vi "utility_edit_device_tree_items_02_01.vi"() -> ()   [LabVIEW 2015]
panel:
  in  "device tree":string[](tree)=["FCXF-X-03-S05"] caption="设备列表"
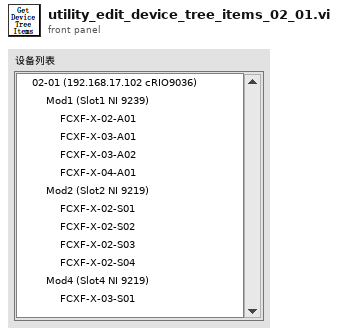
[diagram p1: front panel]
types:
  T1 = enum16{"open", "replace", "create", "open or create", "replace or create", "replace or create with confirmation"}
  T2 = cluster{"Left Cell String":string, "Child Text":string[], "Child Tag":string, "Item Indent":i32, "Child Only?":bool, "Glyph Index":i32}
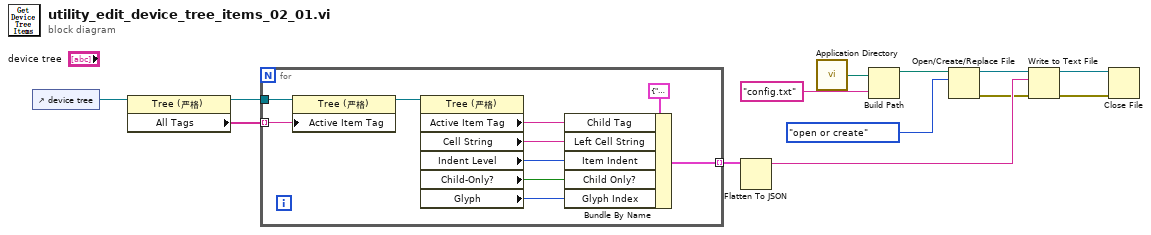
[diagram p0: block diagram]
diagram:
  n1 = control-ref of="device tree"() -> (w13:refnum<vi>)
  n2 = property class="Tree (严格)"(reference=w13) -> (reference out=w12:refnum<vi>, "All Tags"=w11:string[])  [unwired: 1 in, 1 out]
  n3 = for {
    tunnel: w12 -> [w23]
    tunnel: w11 -> [w21] mode=indexing
    tunnel: [w14] -> w10 mode=indexing
    n4 = property class="Tree (严格)"(reference=w23, "Active Item Tag"=w21) -> (reference out=w22:refnum<vi>)  [unwired: 1 in, 1 out]
    n5 = property class="Tree (严格)"(reference=w22) -> ("Active Item Tag"=w19:string, "Cell String"=w18:string, "Indent Level"=w17:i32, "Child-Only?"=w16:bool, "Glyph"=w15:i32)  [unwired: 1 in, 2 out]
    n6 = Bundle By Name(cluster=T2 {"Left Cell String"="FCXF-X-03-T02", "Child Text"=[], "Child Tag"="FCXF-X-03-T02", "Item Indent"=2, "Child Only?"=TRUE, "Glyph Index"=4} ("Item"), "Child Tag"=w19, "Left Cell String"=w18, "Item Indent"=w17, "Child Only?"=w16, "Glyph Index"=w15) -> (w14:T2)
  }
  n7 = Flatten To JSON(anything=w10) -> (JSON string=w9:string)  [unwired: 2 in, 1 out]
  n8 = call <vilib>:"Application Directory.vi"() -> ("Application Directory"=w4:path)
  n9 = Build Path(base path=w4, name or relative path="config.txt" ("名称或相对路径")) -> (appended path=w2:path)
  n10 = Open/Create/Replace File(file path (use dialog)=w2, operation (0:open)=T1."open or create" ("操作(0:open)")) -> (refnum out=w8:refnum<file>, error out=w6:errorcluster)  [unwired: 4 in, 1 out]
  n11 = Write to Text File(file (use dialog)=w8, text=w9, error in=w6) -> (refnum out=w7:refnum<file>, error out=w5:errorcluster)  [unwired: 1 in, 1 out]
  n12 = Close File(refnum=w7, error in=w5) -> ()  [unwired: 2 out]
